vi "getLastSended.vi"(7 "existe archivo":bool, 8 "error in":errorcluster, 10 "tdms file":refnum<k34>) -> (0 "error out":errorcluster, 1 "grupo 3":i32, 2 "grupo 2":i32, 3 "grupo 1":i32)   [LabVIEW 2015]
panel:
  out "transposed array":i32[][](array[numeric])
  out "property value":i64
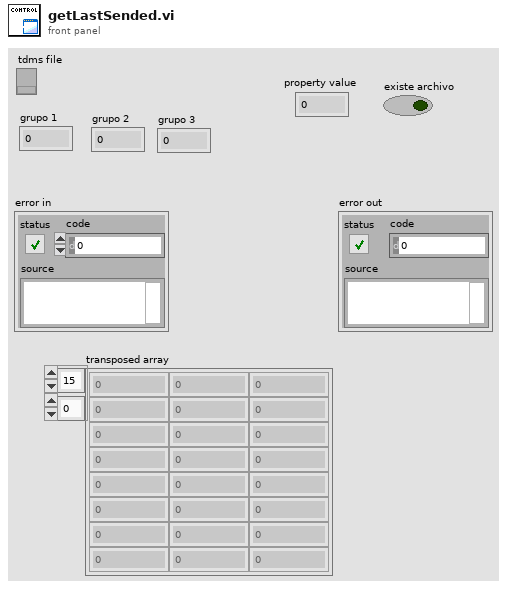
[diagram p1: front panel]
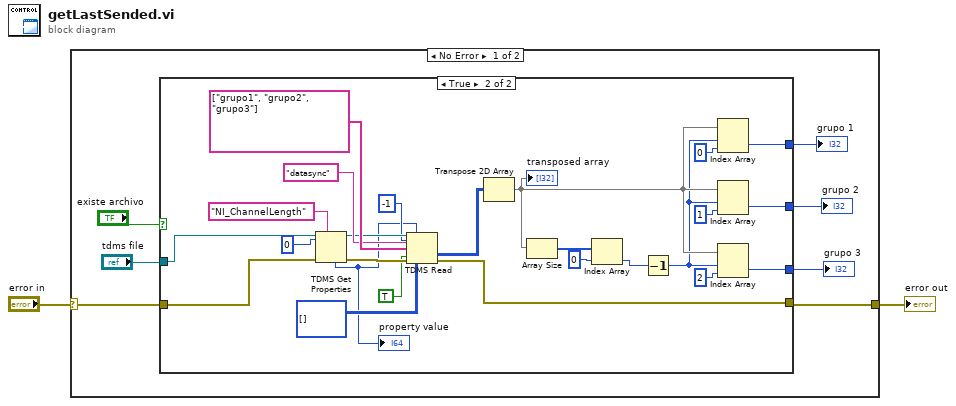
[diagram p0: block diagram]
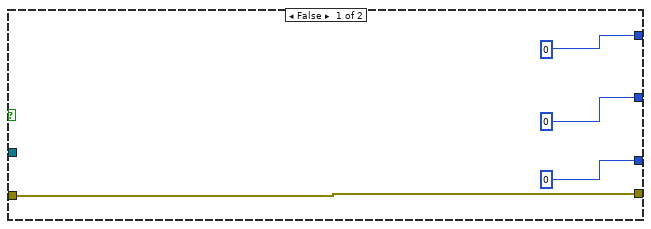
[diagram p2: hidden frame]
diagram:
  n1 = case shown="No Error" "error in" {
    selector: "error in" -> [w5 w39]
    tunnel: [w4 w39] -> w1
    frame No Error {
      n2 = case shown="True" "existe archivo" {
        tunnel: w5 -> [w13 w36]
        tunnel: "tdms file" -> [_ w17]
        tunnel: [w13 w33] -> w4
        tunnel: [0 w28] -> w8
        tunnel: [0 w26] -> w7
        tunnel: [0 w24] -> w6
        frame False {
        }
        frame True {
          n3 = TDMS Get Properties(5:i64 0, 7:"NI_ChannelLength" ("property name"), 8:w36, 11:w17) -> (0:w34:errorcluster, 3:w23:refnum<k34>, 4:w14:i64)  [unwired: 2 in, 3 out]
          "property value" <- w14
          n4 = TDMS Read(0:w23, 1:w14, 2:i64 -1 ("count (-1: all)"), 5:"datasync" ("group name in"), 7:string[] ["grupo1", "grupo2", "grupo3"], 11:w34, 12:i32[][] [], 13:TRUE ("return channels in file order? (F)")) -> (10:w30:i32[][], 15:w33:errorcluster)  [unwired: 4 out]
          n5 = Transpose 2D Array(2D array=w30) -> (transposed array=w20:i32[][])
          "transposed array" <- w20
          n6 = Array Size(array=w20) -> (size(s)=w19:i32[])
          n7 = Index Array(array=w19, index=0) -> (element=w16:i32)
          n8 = Decrement(x=w16) -> (x-1=w15:i32)
          n9 = Index Array(array=w20, index (row)=w15, index (col)=0 ("disabled index (col)")) -> (element=w28:i32)
          n10 = Index Array(array=w20, index (row)=w15, index (col)=1) -> (element=w26:i32)
          n11 = Index Array(array=w20, index (row)=w15, index (col)=2 ("disabled index (col)")) -> (element=w24:i32)
        }
      }
      "grupo 1" <- w8
      "grupo 2" <- w7
      "grupo 3" <- w6
    }
    frame Error {
    }
  }
  "error out" <- w1
